vi "CallEditVI.vi"(8 "VI引用句柄":refnum<vi>, 10 "索引":i32, 11 "TreeControl输入":refnum<vi>) -> (2 "索引输出":i32, 3 "TreeControl输出":refnum<vi>)   [LabVIEW 2020, in "Curve Editor.lvlib"]
uses:
  Curve Editor.lvlib
panel:
  # "通过VI引用打开VI，同时传入参数（一个树形引用，一个I32整数）"
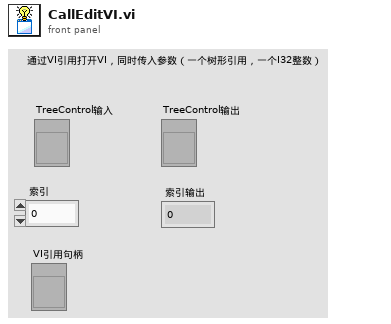
[diagram p1: front panel]
types:
  T1 = enum32{"Invalid", "Standard", "Closed", "Hidden", "Minimized", "Maximized"}
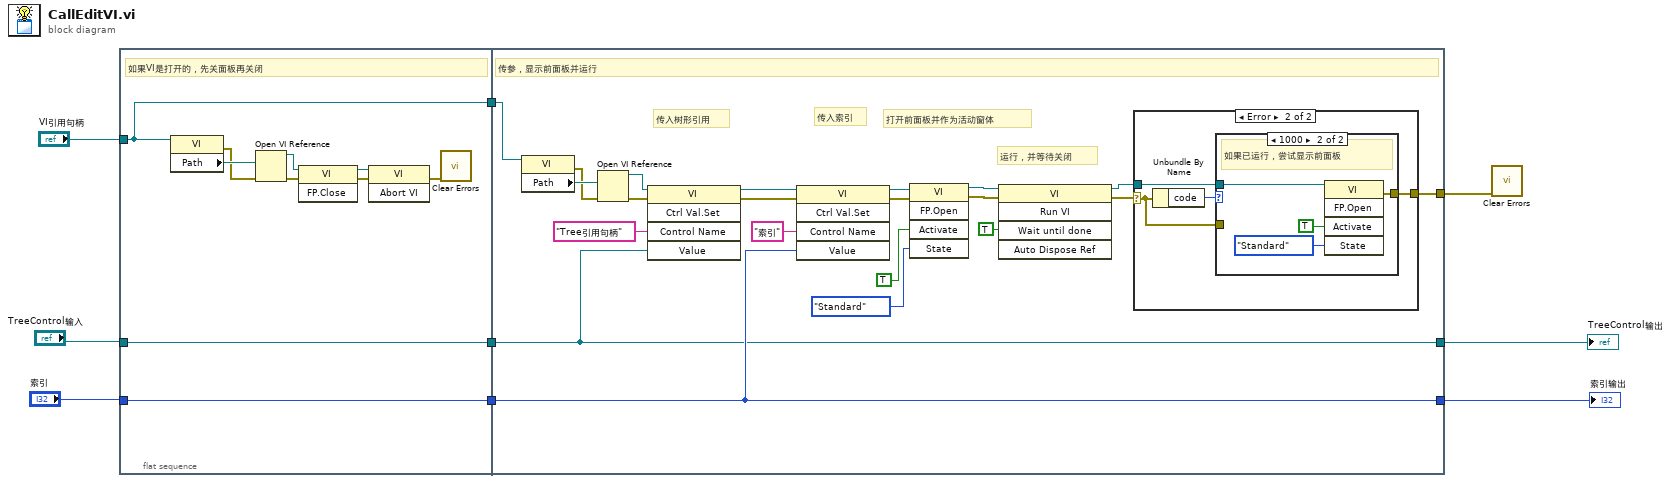
[diagram p0: block diagram]
diagram:
  n1 = flat-sequence {
    tunnel: "索引" -> [w19]
    tunnel: [w19] -> w9
    tunnel: [w12] -> w8
    tunnel: "VI引用句柄" -> [w12]
    tunnel: "TreeControl输入" -> [w11]
    tunnel: [w11] -> w7
    tunnel: w9 -> [w31]
    tunnel: w8 -> [w33]
    tunnel: w7 -> [w30]
    tunnel: [w31] -> w4
    tunnel: [w30] -> w6
    tunnel: [w28] -> w1
    frame #0 {
      # "如果VI是打开的，先关面板再关闭"
      n2 = property class="VI"(reference=w12) -> (error out=w10:errorcluster, "Path"=w13:path)  [unwired: 1 in, 1 out]
      n3 = Open VI Reference(vi path=w13, error in (no error)=w10) -> (vi reference=w14:refnum<vi>, error out=w15:errorcluster)  [unwired: 4 in]
      n4 = invoke class="VI" method="FP.Close"(reference=w14, error in=w15) -> (reference out=w16:refnum<vi>, error out=w17:errorcluster)  [unwired: 1 in, 1 out]
      n5 = invoke class="VI" method="Abort VI"(reference=w16, error in=w17) -> (error out=w18:errorcluster)  [unwired: 1 in, 2 out]
      n6 = call <vilib>:"Clear Errors.vi"("error in (no error)"=w18) -> ()  [unwired: 5 in, 2 out]
    }
    frame #1 {
      # "运行，并等待关闭"
      # "打开前面板并作为活动窗体"
      # "传入索引"
      # "传入树形引用"
      # "传参，显示前面板并运行"
      n7 = property class="VI"(reference=w33) -> (error out=w29:errorcluster, "Path"=w40:path)  [unwired: 1 in, 1 out]
      n8 = Open VI Reference(vi path=w40, error in (no error)=w29) -> (vi reference=w39:refnum<vi>, error out=w36:errorcluster)  [unwired: 4 in]
      n9 = invoke class="VI" method="Ctrl Val.Set"(reference=w39, error in=w36, "Control Name"="Tree引用句柄" ("控件名"), "Value"=w30) -> (reference out=w37:refnum<vi>, error out=w35:errorcluster)  [unwired: 1 in, 3 out]
      n10 = invoke class="VI" method="Ctrl Val.Set"(reference=w37, error in=w35, "Control Name"="索引" ("控件名"), "Value"=w31) -> (reference out=w25:refnum<vi>, error out=w24:errorcluster)  [unwired: 1 in, 3 out]
      n11 = invoke class="VI" method="FP.Open"(reference=w25, error in=w24, "Activate"=TRUE ("激活？"), "State"=T1."Standard" ("状态")) -> (reference out=w23:refnum<vi>, error out=w22:errorcluster)  [unwired: 1 in, 3 out]
      n12 = invoke class="VI" method="Run VI"(reference=w23, error in=w22, "Wait until done"=TRUE ("结束前等待")) -> (reference out=w21:refnum<vi>, error out=w20:errorcluster)  [unwired: 2 in, 3 out]
      n13 = case shown="Error" w20 {
        selector: w20 -> [w41 w43]
        tunnel: w21 -> [_ w44]
        tunnel: [w41 w42] -> w28
        frame No Error {
        }
        frame Error {
          n14 = Unbundle By Name(w43) -> ("code"=w45:i32)
          n15 = case shown="1000" w45 {
            tunnel: w44 -> [_ w48]
            tunnel: w43 -> [w46 _]
            tunnel: [w46 w47] -> w42
            frame 0, Default {
            }
            frame 1000 {
              # "如果已运行，尝试显示前面板"
              n16 = invoke class="VI" method="FP.Open"(reference=w48, "Activate"=TRUE ("激活？"), "State"=T1."Standard" ("状态")) -> (error out=w47:errorcluster)  [unwired: 2 in, 4 out]
            }
          }
        }
      }
    }
  }
  n17 = call <vilib>:"Clear Errors.vi"("error in (no error)"=w1) -> ()  [unwired: 5 in, 2 out]
  "索引输出" <- w4
  "TreeControl输出" <- w6
